vi "stylize sequence window.vi"(5 "import style":bool, 7 "use styles":bool, 8 "line #":i32=35, 9 "top row":u16, 10 "commands in styles":T1(array[cluster])=[{"commands"="Run Macro", "Color"=16711680, "Boolean"=TRUE, "Color Box"=0}, {"commands"="SubMacro", "Color"=0, "Boolean"=TRUE, "Color Box"=0}, {"commands"="Set Field", "Color"=16860, "Boolean"=TRUE, "Color Box"=0}, {"commands"="Wait for Temperature", "Color"=0, "Boolean"=TRUE, "Color Box"=0}, {"commands"="Wait for VI value", "Color"=0, "Boolean"=FALSE, "Color Box"=0}, {"commands"="Wait for Field Stable", "Color"=16860, "Boolean"=TRUE, "Color Box"=0}, {"commands"="Set Temperature", "Color"=16860, "Boolean"=TRUE, "Color Box"=0}], 11 "ListBox in":refnum<vi>) -> ()   [LabVIEW 2025]
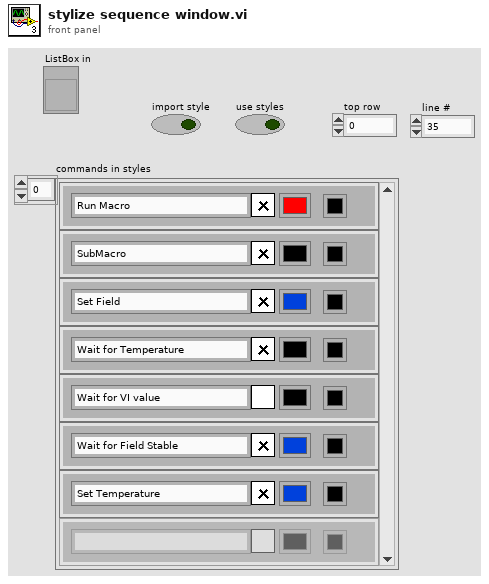
[diagram p1: front panel]
types:
  T1 = cluster{"commands":string, "Color":u32, "Boolean":bool, "Color Box":u32}[]
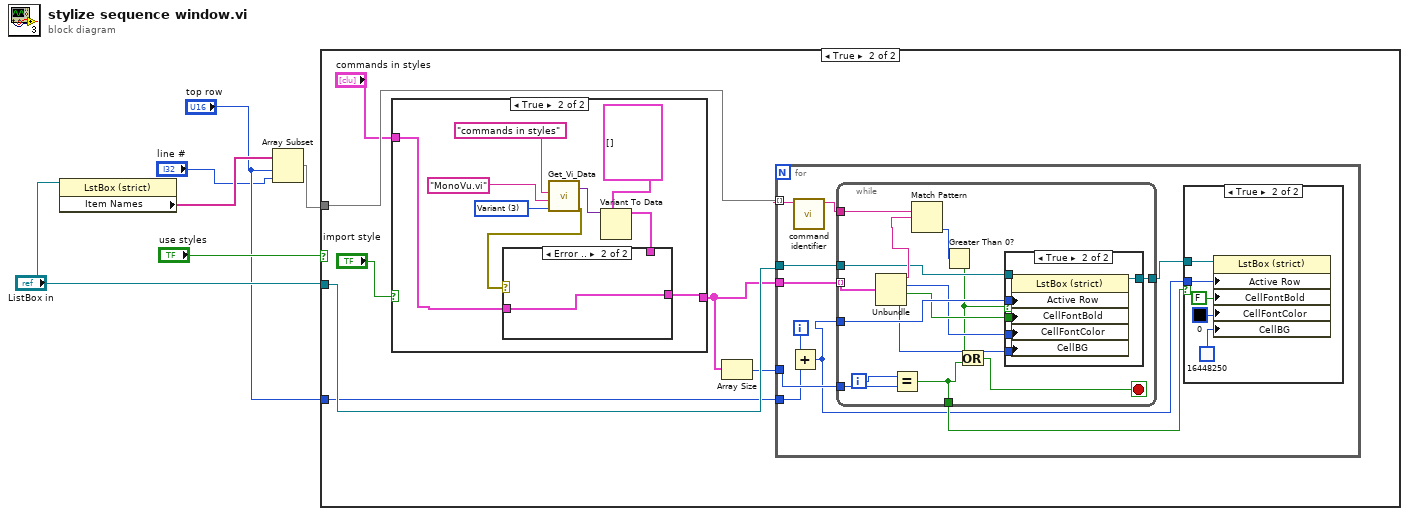
[diagram p0: block diagram]
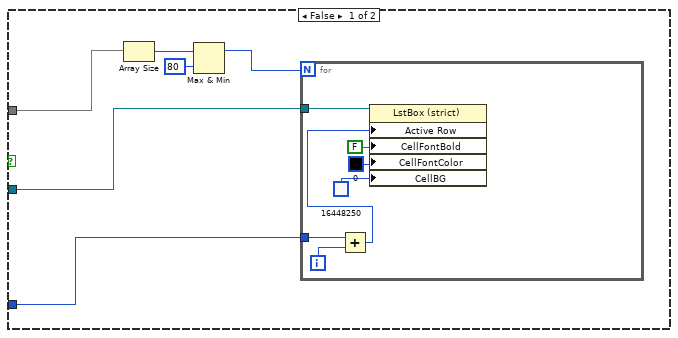
[diagram p2: hidden frame]
diagram:
  n1 = property on="Property Node" class="LstBox (strict)"(reference="ListBox in") -> ("Item Names"=w4:string[])  [unwired: 1 in, 2 out]
  n2 = Array Subset(array=w4, index="top row", length="line #") -> (w3:string[])
  n3 = case shown="True" "use styles" {
    tunnel: w3 -> [w11 w25]
    tunnel: "ListBox in" -> [w12 w24]
    tunnel: "top row" -> [w7 w20]
    frame False {
      n4 = Array Size(array=w11) -> (size(s)=w10:i32)
      n5 = Max & Min(x=w10, y=80) -> (max(x,y)=w9:i32)  [unwired: 1 out]
      n6 = for {
        N: w9 -> [_]
        tunnel: w12 -> [w19]
        tunnel: w7 -> [w14]
        i -> [w15]
        n7 = Add(x=w14, y=w15) -> (x+y=w13:i32)
        n8 = property class="LstBox (strict)"(reference=w19, "Active Row"=w13, "CellFontBold"=FALSE ("Active Row:Cell Font:Bold"), "CellFontColor"=u32 0 ("Active Row:Cell Font:Color"), "CellBG"=u32 16448250 ("Active Row:Cell Font:Color")) -> ()  [unwired: 1 in, 2 out]
      }
    }
    frame True {
      n9 = case shown="True" "import style" {
        tunnel: [w64 w68] -> w23
        tunnel: "commands in styles" -> [w64 w66]
        frame False {
        }
        frame True {
          w73 = u16 3 items=["String", "Double", "Boolean", "Variant"] ("Data Type")
          n10 = call "Get_Vi_Data.vi"("Data Type"=w73, "VI name"="MonoVu.vi", "Control Name"="commands in styles") -> ("error out"=w69:errorcluster, "Data (Variant)"=w70:variant)  [unwired: 4 in, 3 out]
          n11 = Variant To Data(type=T1 [] ("commands in styles 2"), Variant=w70) -> (data=w67:T1)  [unwired: 1 in, 1 out]
          n12 = case shown="Error .." w69 {
            tunnel: [w74 w75] -> w68
            tunnel: w67 -> [w74 _]
            tunnel: w66 -> [_ w75]
            frame No Error {
            }
            frame Error {
            }
          }
        }
      }
      n13 = Array Size(array=w23) -> (size(s)=w22:i32)
      n14 = for {
        tunnel: w25 -> [w36] mode=indexing
        tunnel: w23 -> [w35]
        tunnel: w24 -> [w33]
        tunnel: w22 -> [w30]
        tunnel: w20 -> [w28]
        i -> [w29]
        n15 = Add(x=w29, y=w28) -> (x+y=w27:i32)
        n16 = call "command identifier.vi"("Input command"=w36) -> ("Identifield command"=w34:string)  [unwired: 10 in]
        n17 = while {
          tunnel: w35 -> [w48] mode=indexing
          tunnel: w34 -> [w51]
          tunnel: w27 -> [w49]
          tunnel: w33 -> [w44]
          tunnel: [w43] -> w32
          tunnel: [w40] -> w31
          tunnel: w30 -> [w38]
          i -> [w39]
          stop <- w41 stop-if-true
          n18 = Unbundle(w48) -> ("commands"=w47:string, "Color"=w45:u32, "Boolean"=w46:bool, "Color Box"=w37:u32)
          n19 = Equal?(x=w39, y=w38) -> (x = y?=w40:bool)
          n20 = Match Pattern(string=w51, regular expression=w47) -> (offset past match=w50:i32)  [unwired: 1 in, 3 out]
          n21 = Greater Than 0?(x=w50) -> (x > 0?=w42:bool)
          n22 = Or(x=w42, y=w40) -> (x .or. y?=w41:bool)
          n23 = case shown="True" w42 {
            tunnel: w49 -> [_ w58]
            tunnel: w46 -> [_ w57]
            tunnel: w45 -> [_ w56]
            tunnel: w44 -> [w52 w55]
            tunnel: [w52 w54] -> w43
            tunnel: w37 -> [_ w53]
            frame False {
            }
            frame True {
              n24 = property on="Property Node" class="LstBox (strict)"(reference=w55, "Active Row"=w58, "CellFontBold"=w57, "CellFontColor"=w56, "CellBG"=w53) -> (reference out=w54:refnum<vi>)  [unwired: 1 in, 1 out]
            }
          }
        }
        n25 = case shown="True" w31 {
          tunnel: w27 -> [_ w63]
          tunnel: w32 -> [_ w60]
          frame False {
          }
          frame True {
            n26 = property on="Property Node" class="LstBox (strict)"(reference=w60, "Active Row"=w63, "CellFontBold"=FALSE ("Active Row:Cell Font:Bold"), "CellFontColor"=u32 0 ("Active Row:Cell Font:Color"), "CellBG"=u32 16448250 ("Active Row:Cell Font:Color")) -> ()  [unwired: 1 in, 2 out]
          }
        }
      }
    }
  }
